vi "Get VI Printing Options.vi"(8 "error in (no error)":errorcluster, 11 "VI Refnum":refnum<vi>) -> (0 "error out":errorcluster, 1 "orientation (unchanged)":T7 items=["Unchanged", "portrait", "landscape"], 2 "panel scaling for page (unchanged)":T8 items=["Unchanged", "No Scaling", "Scale front panel to fit"], 3 "VI Refnum out":refnum<vi>, 4 "margins":T4={"override VI margins (false)"=FALSE, "margins (1.00)"={"top"=1.0, "left"=1.0, "right"=1.0, "bottom"=1.0}, "measurement system (default)"=0} {"measurement system (default)" items=["Default", "US", "Metric"]; "margins (1.00)"."right" format="%.2f"; "margins (1.00)"."bottom" format="%.2f"; "margins (1.00)"."top" format="%.2f"; "margins (1.00)"."left" format="%.2f"}, 5 "page header options":T1={"page headers (unchanged)"=0, "page header content options"={"Include VI Name"=TRUE, "Include VI Path"=TRUE, "Include Last Modification Date"=TRUE, "Include Date Printed"=TRUE, "Include Page Number"=TRUE, "Include VI Icon"=TRUE}} {"page headers (unchanged)" items=["Unchanged", "Include page headers", "Do not include page headers"]})   [LabVIEW 2017, in "NI_ReportGenerationCore.lvlib"]
uses:
  <vilib>/Utility/NIReport.llb/NI_ReportGenerationCore.lvlib
  <vilib>/printing/EasyPrintingControls.llb/panel_scaling_for_page.ctl
  <vilib>/printing/EasyPrintingControls.llb/orientation.ctl
  <vilib>/printing/EasyPrintingControls.llb/margins.ctl
  <vilib>/printing/EasyPrintingControls.llb/margin_values.ctl
  <vilib>/printing/EasyPrintingControls.llb/measurement_system.ctl
  <vilib>/printing/EasyPrintingControls.llb/page_header_options.ctl
  <vilib>/printing/EasyPrintingControls.llb/page_headers.ctl
  <vilib>/printing/EasyPrintingControls.llb/page_header_content_options.ctl
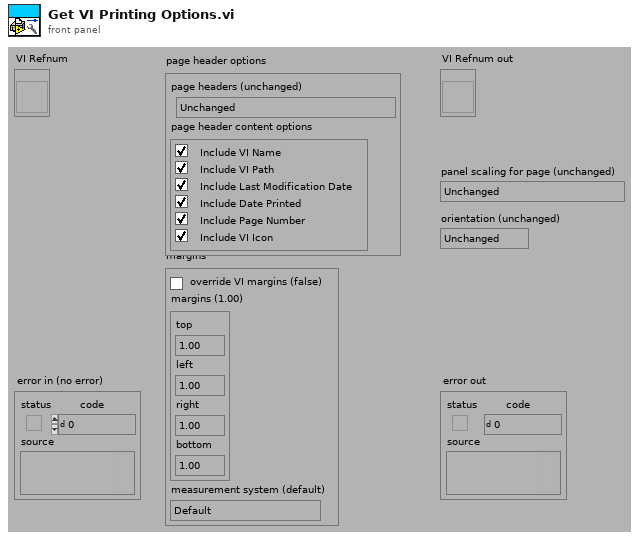
[diagram p1: front panel]
types:
  T1 = typedef "NI_ReportGenerationCore.lvlib/page_header_options.ctl" = cluster{"page headers (unchanged)":T2, "page header content options":T3}
  T2 = typedef "NI_ReportGenerationCore.lvlib/page_headers.ctl" = u16
  T3 = typedef "NI_ReportGenerationCore.lvlib/page_header_content_options.ctl" = cluster{"Include VI Name":bool, "Include VI Path":bool, "Include Last Modification Date":bool, "Include Date Printed":bool, "Include Page Number":bool, "Include VI Icon":bool}
  T4 = typedef "NI_ReportGenerationCore.lvlib/margins.ctl" = cluster{"override VI margins (false)":bool, "margins (1.00)":T5, "measurement system (default)":T6}
  T5 = typedef "NI_ReportGenerationCore.lvlib/margin_values.ctl" = cluster{"top":dbl, "left":dbl, "right":dbl, "bottom":dbl}
  T6 = typedef "NI_ReportGenerationCore.lvlib/measurement_system.ctl" = u16
  T7 = typedef "NI_ReportGenerationCore.lvlib/orientation.ctl" = u16
  T8 = typedef "NI_ReportGenerationCore.lvlib/panel_scaling_for_page.ctl" = u16
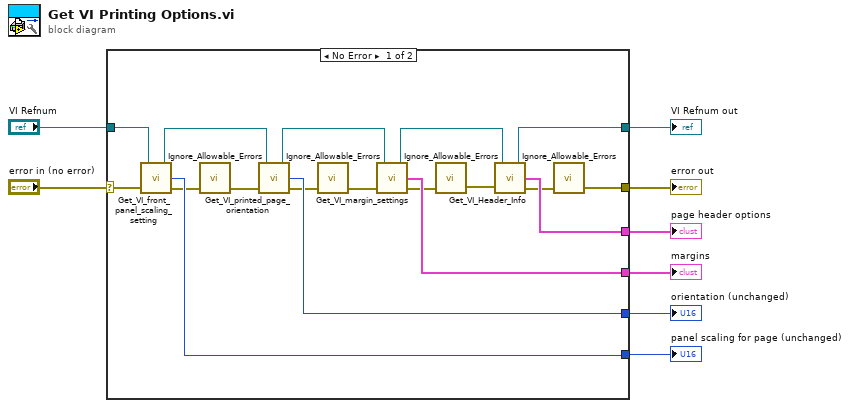
[diagram p0: block diagram]
diagram:
  n1 = case shown="No Error" "error in (no error)" {
    selector: "error in (no error)" -> [w26 w28]
    tunnel: [w14 w28] -> w7
    tunnel: [w9 w27] -> w5
    tunnel: "VI Refnum" -> [w13 w27]
    tunnel: [w25 _] -> w4
    tunnel: [w24 _] -> w3
    tunnel: [w23 _] -> w2
    tunnel: [w22 _] -> w1
    frame No Error {
      n2 = call <vilib>:"Get_VI_front_panel_scaling_setting.vi"("reference"=w13, "error in (no error)"=w26) -> ("reference out"=w12:refnum<vi>, "scaling"=w25:T8, "error out"=w21:errorcluster)
      n3 = call <vilib>:"Ignore_Allowable_Errors.vi"("error in (no error)"=w21) -> ("error out"=w20:errorcluster)  [unwired: 10 in]
      n4 = call <vilib>:"Get_VI_printed_page_orientation.vi"("reference in"=w12, "error in (no error)"=w20) -> ("reference out"=w11:refnum<vi>, "Orientaion"=w24:T7, "error out"=w19:errorcluster)
      n5 = call <vilib>:"Ignore_Allowable_Errors.vi"("error in (no error)"=w19) -> ("error out"=w18:errorcluster)  [unwired: 10 in]
      n6 = call <vilib>:"Get_VI_margin_settings.vi"("reference"=w11, "error in (no error)"=w18) -> ("reference out"=w10:refnum<vi>, "Margin"=w23:T4, "error out"=w17:errorcluster)
      n7 = call <vilib>:"Ignore_Allowable_Errors.vi"("error in (no error)"=w17) -> ("error out"=w16:errorcluster)  [unwired: 10 in]
      n8 = call <vilib>:"Get_VI_Header_Info.vi"("reference"=w10, "error in (no error)"=w16) -> ("reference 2"=w9:refnum<vi>, "Header info"=w22:T1, "error out"=w15:errorcluster)
      n9 = call <vilib>:"Ignore_Allowable_Errors.vi"("error in (no error)"=w15) -> ("error out"=w14:errorcluster)  [unwired: 10 in]
    }
    frame Error {
    }
  }
  "error out" <- w7
  "orientation (unchanged)" <- w3
  "panel scaling for page (unchanged)" <- w4
  "margins" <- w2
  "VI Refnum out" <- w5
  "page header options" <- w1
